vi "Config - Load.vi"(8 "error in (no error)":errorcluster, 11 "Config Data":T1) -> (0 "error out":errorcluster, 3 "Config Data":T1)   [LabVIEW 2017]
doc: "Load Configuration parameters from external XML file"
uses:
  Controls/Config Data.ctl
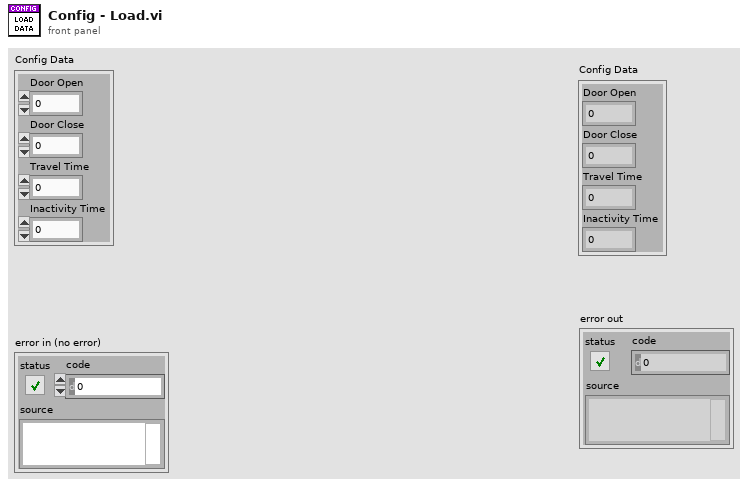
[diagram p1: front panel]
types:
  T1 = typedef "Config Data.ctl" = cluster{"Door Open":dbl, "Door Close":dbl, "Travel Time":dbl, "Inactivity Time":dbl}
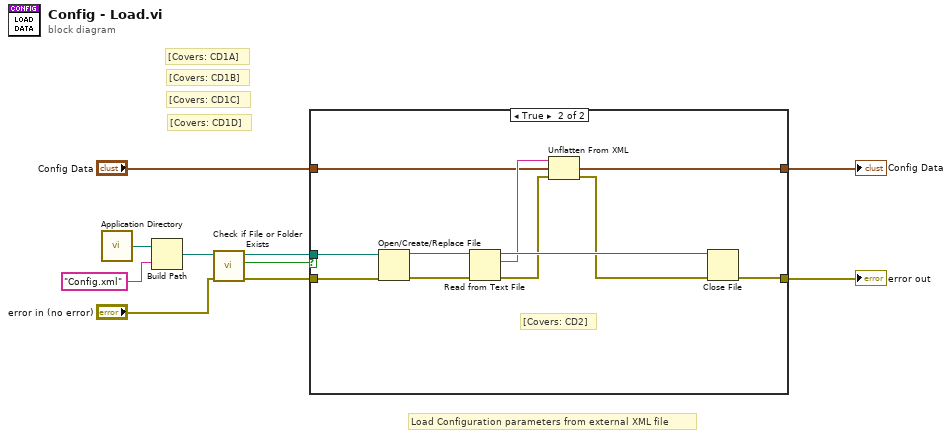
[diagram p0: block diagram]
diagram:
  # "Load Configuration parameters from external XML file"
  # "[Covers: CD1D]"
  # "[Covers: CD1C]"
  # "[Covers: CD1B]"
  # "[Covers: CD1A]"
  n1 = call <vilib>:"Application Directory.vi"() -> ("Application Directory"=w10:path)
  n2 = Build Path(base path=w10, name or relative path="Config.xml") -> (appended path=w8:path)
  n3 = call <vilib>:"Check if File or Folder Exists.vi"("error in (no error)"="error in (no error)", "path"=w8) -> ("error out"=w5:errorcluster, "file or folder exists?"=w7:bool, "dup path"=w6:path)  [unwired: 7 in]
  n4 = case shown="True" w7 {
    tunnel: w6 -> [_ w23]
    tunnel: w5 -> [w12 w22]
    tunnel: [w12 w13] -> w1
    tunnel: "Config Data" -> [w11 w16]
    tunnel: [w11 w15] -> w2
    frame False {
      # "#TODO\nCreate new config file\nand write default values"
      # "[Covers: CD3]"
    }
    frame True {
      # "[Covers: CD2]"
      n5 = Open/Create/Replace File(file path (use dialog)=w23, error in=w22) -> (refnum out=w20:refnum<file>, error out=w21:errorcluster)  [unwired: 4 in, 1 out]
      n6 = Read from Text File(file (use dialog)=w20, error in=w21) -> (refnum out=w19:refnum<file>, text=w17:string, error out=w18:errorcluster)  [unwired: 2 in, 1 out]
      n7 = Unflatten From XML(xml string=w17, type=w16, error in (no error)=w18) -> (value=w15:T1, error out=w14:errorcluster)
      n8 = Close File(refnum=w19, error in=w14) -> (error out=w13:errorcluster)  [unwired: 1 out]
    }
  }
  "Config Data" <- w2
  "error out" <- w1
